vi "(SubVI) Correct the center when oneside is exceeded.vi"(0 "initial position (um)":dbl, 1 "maxQPD position (um)":dbl, 3 "Guess center (um)":dbl, 4 "minQPD position (um)":dbl, 5 "range (um)":dbl) -> (7 "Correct center (um)":dbl)   [LabVIEW 2014]
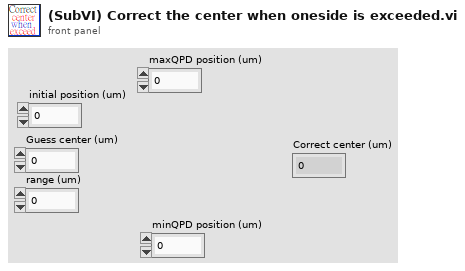
[diagram p1: front panel]
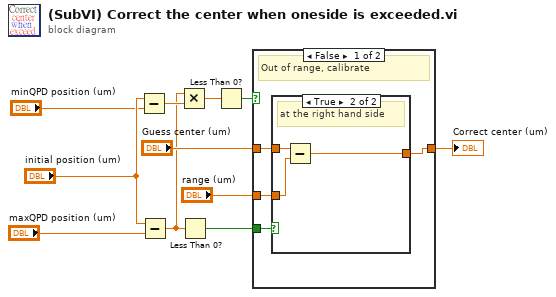
[diagram p0: block diagram]
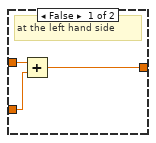
[diagram p2: hidden frame]
diagram:
  n1 = Subtract(x="initial position (um)", y="minQPD position (um)") -> (x-y=w8:dbl)
  n2 = Subtract(x="initial position (um)", y="maxQPD position (um)") -> (x-y=w3:dbl)
  n3 = Multiply(x=w3, y=w8) -> (x*y=w7:dbl)
  n4 = Less Than 0?(x=w3) -> (x < 0?=w2:bool)
  n5 = Less Than 0?(x=w7) -> (x < 0?=w6:bool)
  n6 = case shown="False" w6 {
    tunnel: [w12 w22] -> w5
    tunnel: "Guess center (um)" -> [w14 w22]
    tunnel: w2 -> [w15 _]
    tunnel: "range (um)" -> [w13 _]
    frame False {
      # "Out of range, calibrate"
      n7 = case shown="True" w15 {
        tunnel: w14 -> [w18 w21]
        tunnel: w13 -> [w17 w20]
        tunnel: [w16 w19] -> w12
        frame False {
          # "at the left hand side"
          n8 = Add(x=w18, y=w17) -> (x+y=w16:dbl)
        }
        frame True {
          # "at the right hand side"
          n9 = Subtract(x=w21, y=w20) -> (x-y=w19:dbl)
        }
      }
    }
    frame True {
      # "correct center"
    }
  }
  "Correct center (um)" <- w5
